vi "EminemExecuteLogic.vi"(9 "Feed_Vel_RPM":dbl, 10 "Shooter_Bottom_Vel_RPM":dbl, 11 "Shooter_Top_Vel_RPM":dbl) -> (0 "Box states":T1=enum."13-AmpDone", 1 "Shooter_Feed_Motor_Out":dbl, 2 "Shooter_Bottom_Motor_Out":dbl, 3 "Shooter_Top_Motor_Out":dbl)   [LabVIEW 2023]
uses:
  EminemStatesEnum.ctl
  <vilib>/Rock Robotics/WPI/ThirdParty/JAS_Junk/TrajLib/Trajectory_Library.lvlib
  <vilib>/Rock Robotics/WPI/ThirdParty/JAS_Junk/TrajLib/TypeDef/PID_ERROR_TOLERANCE.ctl
  EminemGlobals.vi
  <vilib>/Rock Robotics/WPI/ThirdParty/JAS_Junk/TrajLib/LinearFilter_MovingAvg_Execute.vi
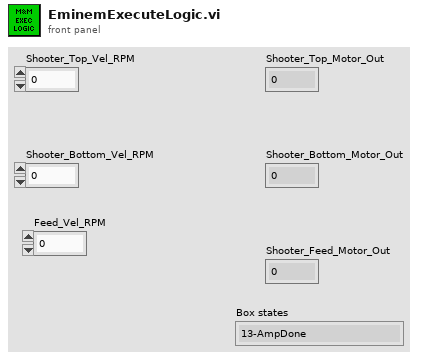
[diagram p1: front panel]
types:
  T1 = typedef "EminemStatesEnum.ctl" = enum16{"0-Init", "1-WaitForCmd", "2-Cancel", "3-ShootStart", "4-ShootRev", "5-RevUpStart", "6-ShootStartFeed&Timer", "7-ShootTimerOrSensorDone", "8-ShootDone", "9-AmpStart", "10-AmpUpToSpd?", "11-AmpStartFeed&Timer", "12-AmpTimerOrSensorDone", "13-AmpDone", "14-RevUpGetCmd"}
  T2 = typedef "Trajectory_Library.lvlib/PID_ERROR_TOLERANCE.ctl" = cluster{"PositionTolerance":dbl, "VelocityTolerance":dbl}
  T3 = enum16{"Moving Average", "Low Pass 1st Order Butterworth", "Low Pass 2nd Order Butterworth", "High Pass 1st Order Butterworth", "High Pass 2nd Order Butterworth"}
  T4 = typedef "Trajectory_Library.lvlib/SIMPLE_MOTOR_FF.ctl" = cluster{"Ks":dbl, "Kv":dbl, "Ka":dbl, "KnInv":dbl}
  T5 = typedef "Trajectory_Library.lvlib/PID_ADV_TUNING.ctl" = cluster{"Kf":dbl, "Kp":dbl, "Ki":dbl, "Kd":dbl, "MaximumIntegral":dbl, "MinimumIntegral":dbl, "Filter Derivative":bool, "IntegralZone":dbl}
  T6 = typedef "Trajectory_Library.lvlib/PID_ADV_LIMITS.ctl" = cluster{"MaxInput":dbl, "MinInput":dbl, "Continuous":bool, "MaxOutput":dbl, "MinOutput":dbl}
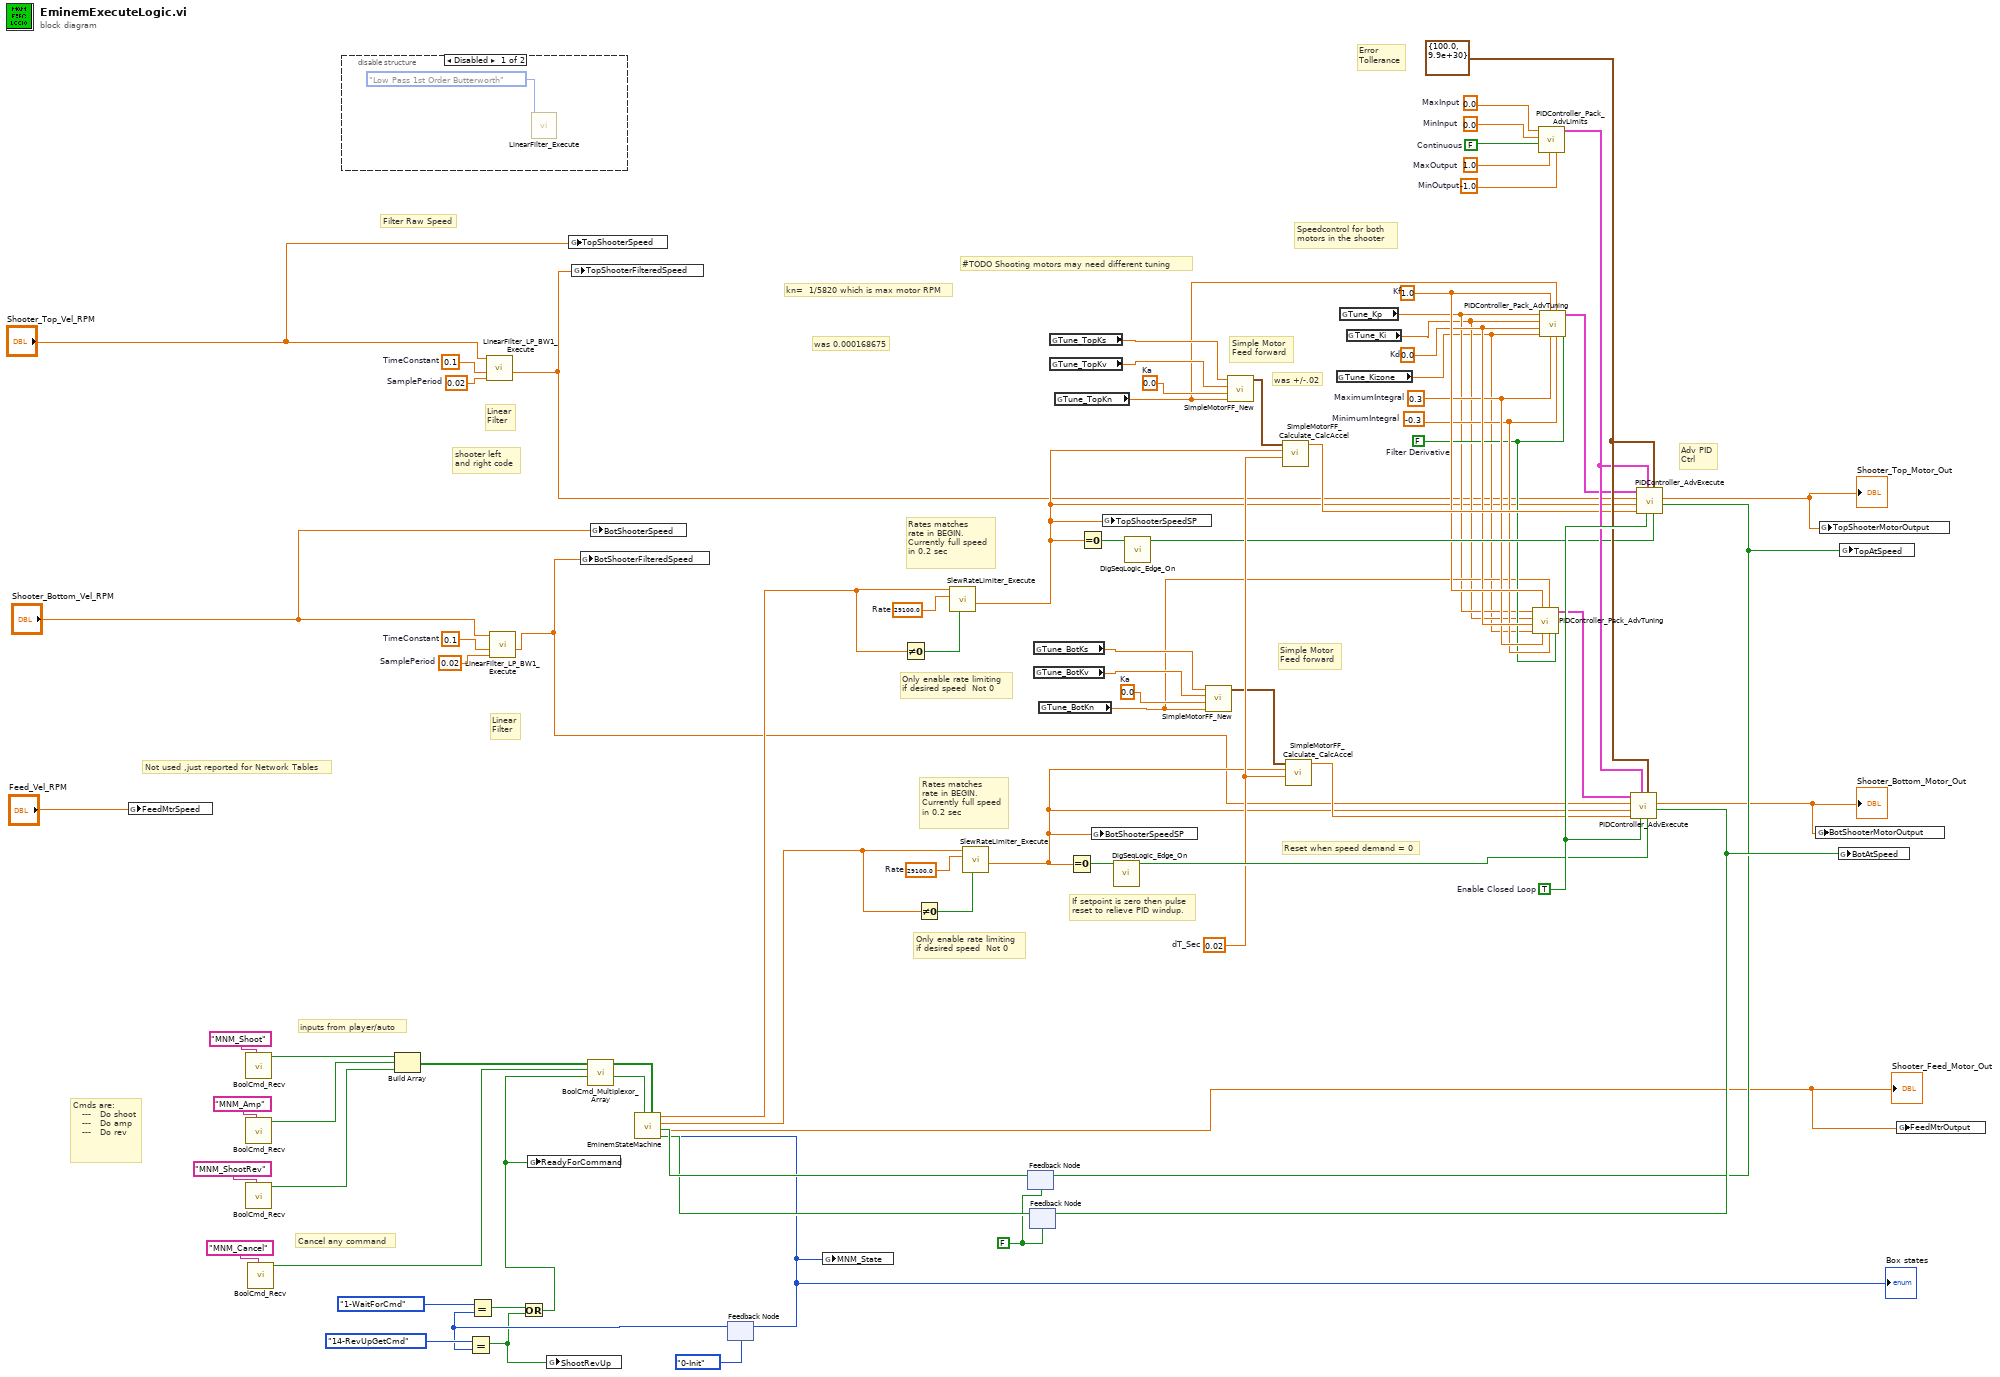
[diagram p0: block diagram]
diagram:
  w27 = 0.0  # Ka
  w34 = FALSE ("AtSetpoint")
  w46 = 29100.0  # Rate
  w77 = 29100.0  # Rate
  w8 = 0.02  # SamplePeriod
  w7 = 0.1  # TimeConstant
  w3 = 0.02  # SamplePeriod
  w2 = 0.1  # TimeConstant
  w79 = TRUE  # Enable Closed Loop
  w73 = T2 {"PositionTolerance"=100.0, "VelocityTolerance"=9.9e+30} ("PID Error Tolerance")
  w68 = 0.0  # Ka
  w23 = 0.0  # Kd
  w24 = 1.0  # Kf
  w22 = 0.3  # MaximumIntegral
  w21 = -0.3  # MinimumIntegral
  w20 = FALSE  # Filter Derivative
  w64 = 0.0  # MinInput
  w65 = FALSE  # Continuous
  w66 = 1.0  # MaxOutput
  w67 = -1.0  # MinOutput
  w63 = 0.0  # MaxInput
  w69 = 0.02  # dT_Sec
  # "Simple Motor\nFeed forward"
  # "was 0.000168675"
  # "#TODO Shooting motors may need different tuning"
  # "Not used ,just reported for Network Tables"
  # "Cmds are:\n   ---   Do shoot\n   ---   Do amp\n   ---   Do rev"
  # "Error \nTollerance"
  # "Filter Raw Speed"
  # "Rates matches\nrate in BEGIN.  \nCurrently full speed\nin 0.2 sec"
  # "Only enable rate limiting\nif desired speed  Not 0"
  # "Reset when speed demand = 0"
  # "was +/-.02"
  # "If setpoint is zero then pulse\nreset to relieve PID windup."
  # "Rates matches\nrate in BEGIN.  \nCurrently full speed\nin 0.2 sec"
  # "Only enable rate limiting\nif desired speed  Not 0"
  # "inputs from player/auto"
  # "Linear\nFilter"
  # "Linear\nFilter"
  # "Speedcontrol for both \nmotors in the shooter"
  # "Simple Motor\nFeed forward"
  # "Adv PID\nCtrl"
  # "Cancel any command"
  # "kn=  1/5820 which is max motor RPM"
  # "shooter left \nand right code"
  n1 = global write "EminemGlobals.vi" "FeedMtrSpeed"("Feed_Vel_RPM") -> ()
  n2 = call <vilib>:"BoolCmd_Recv.vi"("Command Name"="MNM_Shoot") -> ("New Request"=w56:bool)  [unwired: 9 in, 1 out]
  n3 = call <vilib>:"BoolCmd_Recv.vi"("Command Name"="MNM_Amp") -> ("New Request"=w55:bool)  [unwired: 9 in, 1 out]
  n4 = call <vilib>:"BoolCmd_Recv.vi"("Command Name"="MNM_ShootRev") -> ("New Request"=w53:bool)  [unwired: 9 in, 1 out]
  n5 = call <vilib>:"BoolCmd_Recv.vi"("Command Name"="MNM_Cancel") -> ("New Request"=w58:bool)  [unwired: 9 in, 1 out]
  n6 = disable-structure shown="Disabled" {
    frame Disabled {
      n7 = call-poly <vilib>:"LinearFilter_Execute.vi"("Samples"=T3."Low Pass 1st Order Butterworth" ("Filter Type")) -> ()  [unwired: 10 in, 1 out]
    }
    frame Enabled {
    }
  }
  n8 = Build Array(w56, w55, w53) -> (w57:bool[])
  n9 = call <vilib>:"LinearFilter_LP_BW1_Execute.vi"("SamplePeriod"=w8, "TimeConstant"=w7, "Input"="Shooter_Top_Vel_RPM") -> ("Output"=w5:dbl)  [unwired: 8 in]
  n10 = call <vilib>:"LinearFilter_LP_BW1_Execute.vi"("SamplePeriod"=w3, "TimeConstant"=w2, "Input"="Shooter_Bottom_Vel_RPM") -> ("Output"=w4:dbl)  [unwired: 8 in]
  n11 = global write "EminemGlobals.vi" "TopShooterSpeed"("Shooter_Top_Vel_RPM") -> ()
  n12 = global write "EminemGlobals.vi" "TopShooterFilteredSpeed"(w5) -> ()
  n13 = global write "EminemGlobals.vi" "BotShooterFilteredSpeed"(w4) -> ()
  n14 = global write "EminemGlobals.vi" "BotShooterSpeed"("Shooter_Bottom_Vel_RPM") -> ()
  n15 = feedback #1(EminemStatesEnum."0-Init" ("Box states")) -> (w31:T1)
  n16 = Equal?(x=EminemStatesEnum."14-RevUpGetCmd" ("Box states"), y=w31) -> (x = y?=w28:bool)
  n17 = Equal?(x=EminemStatesEnum."1-WaitForCmd" ("Box states"), y=w31) -> (x = y?=w30:bool)
  n18 = Or(x=w30, y=w28) -> (x .or. y?=w29:bool)
  n19 = global write "EminemGlobals.vi" "ReadyForCommand"(w29) -> ()
  n20 = global write "EminemGlobals.vi" "ShootRevUp"(w28) -> ()
  n21 = call <vilib>:"BoolCmd_Multiplexor_Array.vi"("Ready"=w29, "Command Cancel"=w58, "Commands"=w57) -> ("Do Cancel"=w49:bool, "Do Command"=w50:bool[])  [unwired: 7 in]
  n22 = feedback #2(w34) -> (w45:bool)
  n23 = feedback #3(w34) -> (w44:bool)
  n24 = call "EminemStateMachine.vi"("EminemCommand"=w50, "EminemCancel"=w49, "LowerShoot_At_Speed"=w44, "UpperShoot_At_Speed"=w45) -> ("Box states"=w41:T1, "AmpAndFeed-MotorDmd"=w36:dbl, "LowerShooter-RPM_Dmd"=w43:dbl, "UpperShooterAndAmp-RPM_Dmd"=w42:dbl)  [unwired: 4 in]
  "Shooter_Feed_Motor_Out" <- w36
  "Box states" <- w41
  n25 = feedback-in #1(w41) -> ()
  n26 = global write "EminemGlobals.vi" "MNM_State"(w41) -> ()
  n27 = Not Equal To 0?(x=w42) -> (x != 0?=w47:bool)
  n28 = Not Equal To 0?(x=w43) -> (x != 0?=w78:bool)
  n29 = call <vilib>:"SlewRateLimiter_Execute.vi"("Enable"=w47, "PositiveRate"=w46, "Input"=w42) -> ("Output"=w10:dbl)  [unwired: 7 in, 1 out]
  n30 = call <vilib>:"SlewRateLimiter_Execute.vi"("Enable"=w78, "PositiveRate"=w77, "Input"=w43) -> ("Output"=w9:dbl)  [unwired: 7 in, 1 out]
  n31 = global read "EminemGlobals.vi" "Tune_BotKs"() -> (w16:dbl)
  n32 = global read "EminemGlobals.vi" "Tune_BotKv"() -> (w15:dbl)
  n33 = global read "EminemGlobals.vi" "Tune_BotKn"() -> (w14:dbl)
  n34 = global read "EminemGlobals.vi" "Tune_TopKs"() -> (w19:dbl)
  n35 = global read "EminemGlobals.vi" "Tune_TopKv"() -> (w18:dbl)
  n36 = global read "EminemGlobals.vi" "Tune_TopKn"() -> (w17:dbl)
  n37 = Equal To 0?(x=w9) -> (x = 0?=w75:bool)
  n38 = Equal To 0?(x=w10) -> (x = 0?=w52:bool)
  n39 = global write "EminemGlobals.vi" "BotShooterSpeedSP"(w9) -> ()
  n40 = global write "EminemGlobals.vi" "TopShooterSpeedSP"(w10) -> ()
  n41 = call <vilib>:"DigSeqLogic_Edge_On.vi"("Input"=w75) -> ("On Edge"=w76:bool)  [unwired: 10 in]
  n42 = call <vilib>:"DigSeqLogic_Edge_On.vi"("Input"=w52) -> ("On Edge"=w51:bool)  [unwired: 10 in]
  n43 = call <vilib>:"SimpleMotorFF_New.vi"("Kn"=w14, "Ka"=w27, "Kv"=w15, "Ks"=w16) -> ("SIMPLE_MOTOR_FF"=w26:T4)  [unwired: 7 in]
  n44 = call <vilib>:"SimpleMotorFF_New.vi"("Kn"=w17, "Ka"=w68, "Kv"=w18, "Ks"=w19) -> ("SIMPLE_MOTOR_FF"=w70:T4)  [unwired: 7 in]
  n45 = call <vilib>:"SimpleMotorFF_Calculate_CalcAccel.vi"("dT_Sec"=w69, "VelSp"=w10, "SIMPLE_MOTOR_FF"=w70) -> ("FeedForward"=w62:dbl)  [unwired: 8 in]
  n46 = call <vilib>:"SimpleMotorFF_Calculate_CalcAccel.vi"("dT_Sec"=w69, "VelSp"=w9, "SIMPLE_MOTOR_FF"=w26) -> ("FeedForward"=w74:dbl)  [unwired: 8 in]
  n47 = global read "EminemGlobals.vi" "Tune_Kizone"() -> (w11:dbl)
  n48 = global read "EminemGlobals.vi" "Tune_Kp"() -> (w13:dbl)
  n49 = global read "EminemGlobals.vi" "Tune_Ki"() -> (w12:dbl)
  n50 = call <vilib>:"PIDController_Pack_AdvTuning.vi"("Filter Derivative"=w20, "MinimumIntegral"=w21, "Kn"=w14, "MaximumIntegral"=w22, "Kf"=w24, "IntegralZone"=w11, "Kd"=w23, "Ki"=w12, "Kp"=w13) -> ("Adv PID Tuning"=w25:T5)  [unwired: 2 in]
  n51 = call <vilib>:"PIDController_Pack_AdvLimits.vi"("MinOutput"=w67, "MaxOutput"=w66, "Continuous"=w65, "MinInput"=w64, "MaxInput"=w63) -> ("Adv PID Limits"=w72:T6)  [unwired: 6 in]
  n52 = call <vilib>:"PIDController_Pack_AdvTuning.vi"("Filter Derivative"=w20, "MinimumIntegral"=w21, "Kn"=w17, "MaximumIntegral"=w22, "Kf"=w24, "IntegralZone"=w11, "Kd"=w23, "Ki"=w12, "Kp"=w13) -> ("Adv PID Tuning"=w71:T5)  [unwired: 2 in]
  n53 = call <vilib>:"PIDController_AdvExecute.vi"("Reset"=w76, "PID Error Tolerance"=w73, "Auto"=w79, "Adv PID Limits"=w72, "FF-FeedForward"=w74, "SP-SetPoint"=w9, "PV-Measurement"=w4, "Adv PID Tuning"=w25) -> ("AtSetpoint"=w40:bool, "CO-ControlOutput"=w37:dbl)  [unwired: 1 in, 1 out]
  "Shooter_Bottom_Motor_Out" <- w37
  n54 = feedback-in #3(w40) -> ()
  n55 = call <vilib>:"PIDController_AdvExecute.vi"("Reset"=w51, "PID Error Tolerance"=w73, "Auto"=w79, "Adv PID Limits"=w72, "FF-FeedForward"=w62, "SP-SetPoint"=w10, "PV-Measurement"=w5, "Adv PID Tuning"=w71) -> ("AtSetpoint"=w39:bool, "CO-ControlOutput"=w38:dbl)  [unwired: 1 in, 1 out]
  "Shooter_Top_Motor_Out" <- w38
  n56 = feedback-in #2(w39) -> ()
  n57 = global write "EminemGlobals.vi" "BotShooterMotorOutput"(w37) -> ()
  n58 = global write "EminemGlobals.vi" "TopShooterMotorOutput"(w38) -> ()
  n59 = global write "EminemGlobals.vi" "BotAtSpeed"(w40) -> ()
  n60 = global write "EminemGlobals.vi" "TopAtSpeed"(w39) -> ()
  n61 = global write "EminemGlobals.vi" "FeedMtrOutput"(w36) -> ()
